vi "LoadData.vi"   [LabVIEW 2019]
uses:
  20200219Virbtion/Typedef/State.ctl
  LLB/Commonly VI/Ctrl/IDLevel.ctl
  Class/Main Process Class/MPC_VirbVision/Panel RefGlb.vi
  LLB/Commonly VI/Load Glb.vi
types:
  T1 = enum16{"initial", "save", "load", "write", "read"}
  T2 = enum16{"Initial", "Load", "Save", "Read", "WriteSpeed", "WritePoint"}
  T3 = enum8{"Enabled", "Disabled", "Disabled and Grayed Out"}
  T4 = typedef "IDLevel.ctl" = enum16{"Administrator", "Engineer", "Operator", "LogIn/Out"}
  T5 = typedef "State.ctl" = enum16{"Initalize", "Idle", "Update", "Channel1", "Channel2", "Channel3", "Channel4", "Channel1 Sample", "Channel2 Sample", "Channel3 Sample", "Channel4 Sample", "Waveform", "DAQ Rate", "ModelList", "Add", "Remove", "Set Time", "Test", "Start Time", "Check Time", "Save", "Frontward", "Leftward", "Backward", "Rightward", "Stop", "Center", "Bump", "Add Project", "Remove Project", "Project List", "Project Name", "Project OK", "Response", "Exit"}
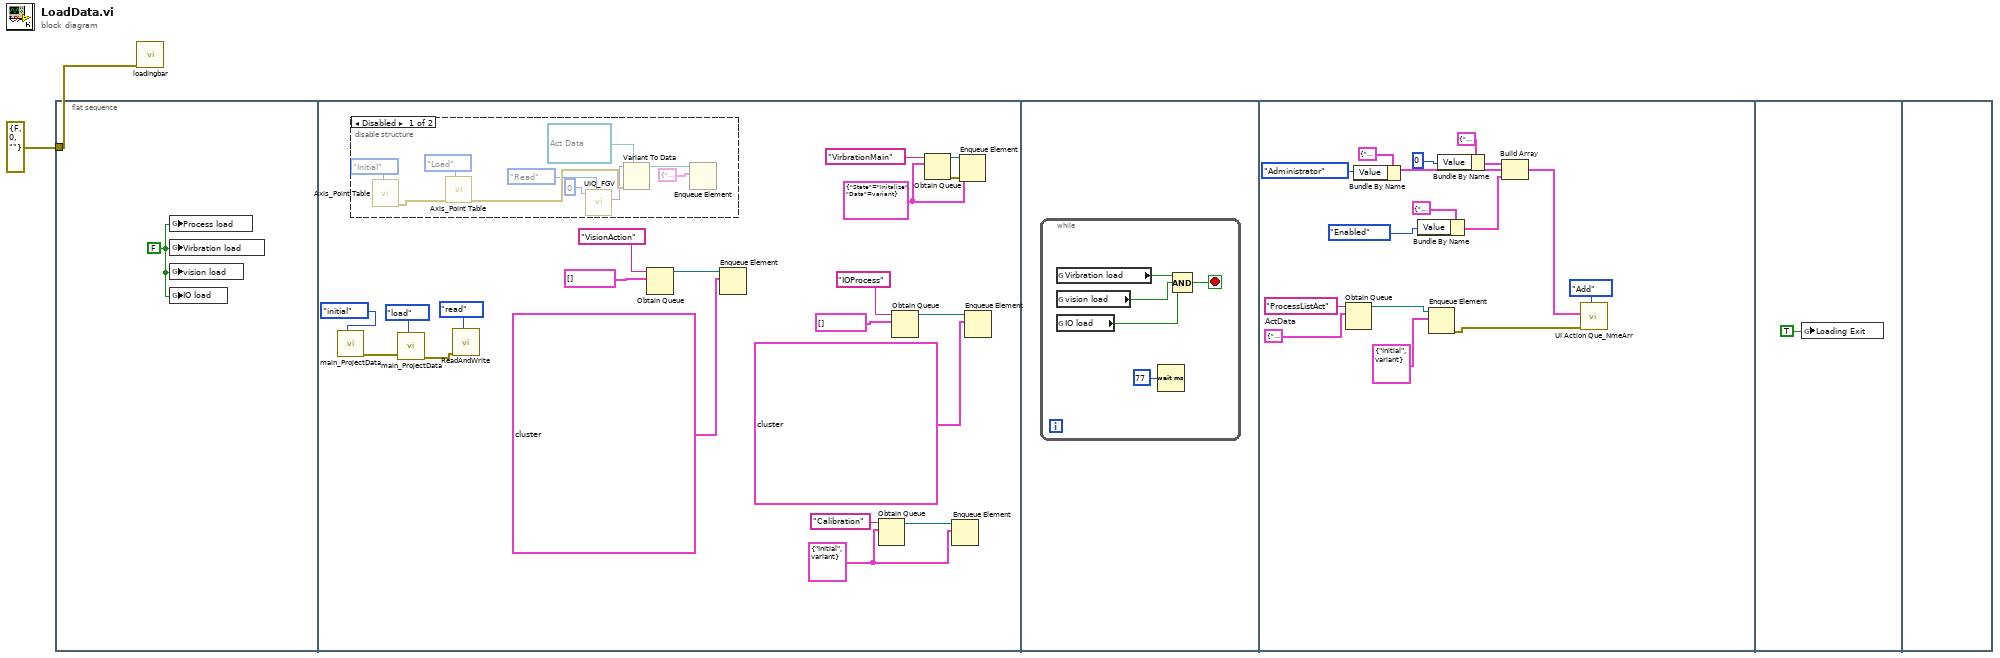
[diagram p0: block diagram]
diagram:
  w1 = errorcluster {"status"=FALSE, "code"=0, "source"=""} ("error constant")
  n1 = flat-sequence {
    tunnel: w1 -> [_]
    frame #0 {
      w2 = FALSE ("IO load")
      n2 = global write "Panel RefGlb.vi" "Process load"(w2) -> ()
      n3 = global write "Panel RefGlb.vi" "Virbration load"(w2) -> ()
      n4 = global write "Panel RefGlb.vi" "vision load"(w2) -> ()
      n5 = global write "Panel RefGlb.vi" "IO load"(w2) -> ()
    }
    frame #1 {
      w19 = cluster{"State":T5, "Data":variant} {"State"=enum."Initalize", "Data"=variant}
      w20 = cluster{"Action":string, "Varient":variant} {"Action"="Initial", "Varient"=variant} ("element")
      n6 = call "main_ProjectData.vi"("Enum"=T1."initial") -> ("error out"=w3:errorcluster)  [unwired: 8 in, 2 out]
      n7 = disable-structure shown="Disabled" {
        frame Disabled {
          n8 = call "Axis_Point Table.vi"("Enum"=T2."Initial") -> ("error Out"=w32:errorcluster)  [unwired: 8 in, 2 out]
          n9 = call "Axis_Point Table.vi"("Enum"=T2."Load", "error In"=w32) -> ("error Out"=w30:errorcluster)  [unwired: 7 in, 2 out]
          n10 = call "UIQ_FGV.vi"("Enum"=enum16{"Initial", "Write", "Read"}."Read", "Index"=0) -> ("DataOut"=w26:variant)  [unwired: 9 in]
          n11 = Variant To Data(error in=w30, type=refnum<queue> refnum ("Axis Q"), Variant=w26) -> (data=w27:refnum<queue>)  [unwired: 1 out]
          n12 = Enqueue Element(queue=w27, element=cluster{"Action":string, "Data":variant} {"Action"="LoadParameter", "Data"=variant}) -> ()  [unwired: 2 in, 3 out]
        }
        frame Enabled {
        }
      }
      n13 = call "main_ProjectData.vi"("Enum"=T1."load", "error in"=w3) -> ("error out"=w7:errorcluster)  [unwired: 7 in, 2 out]
      n14 = call "ReadAndWrite.vi"("Enum"=enum16{"initial", "save", "read"}."read", "error in"=w7) -> ()  [unwired: 9 in, 1 out]
      n15 = Obtain Queue(name (unnamed)="VisionAction", element data type=cluster{"Action":string, "Varient":variant}[] []) -> (queue out=w9:refnum<queue>)  [unwired: 3 in, 2 out]
      n16 = Enqueue Element(queue=w9, element=cluster{"Action":string, "Varient":variant}[] [{"Action"="Get Root Path", "Varient"=variant}, {"Action"="Initial Project", "Varient"=variant}, {"Action"="UpdateProjectSet", "Varient"=variant}, {"Action"="UpDateDataToList ROI", "Varient"=variant}, {"Action"="Initial Camera", "Varient"=variant}, {"Action"="loadfinish", "Varient"=variant}]) -> ()  [unwired: 2 in, 3 out]
      n17 = Obtain Queue(name (unnamed)="Calibration", element data type=w20) -> (queue out=w21:refnum<queue>)  [unwired: 3 in, 2 out]
      n18 = Obtain Queue(name (unnamed)="IOProcess", element data type=cluster{"Action":string, "Varient":variant}[] []) -> (queue out=w13:refnum<queue>)  [unwired: 3 in, 2 out]
      n19 = Obtain Queue(name (unnamed)="VirbrationMain", element data type=w19) -> (queue out=w17:refnum<queue>, error out=w16:errorcluster)  [unwired: 3 in, 1 out]
      n20 = Enqueue Element(queue=w21, element=w20) -> ()  [unwired: 2 in, 3 out]
      n21 = Enqueue Element(queue=w17, element=w19, error in (no error)=w16) -> ()  [unwired: 1 in, 3 out]
      n22 = Enqueue Element(queue=w13, element=cluster{"Action":string, "Varient":variant}[] [{"Action"="Get Root Path", "Varient"=variant}, {"Action"="Initial Project", "Varient"=variant}, {"Action"="UpdateProjectSet", "Varient"=variant}, {"Action"="Initial IOName", "Varient"=variant}, {"Action"="loadfinish", "Varient"=variant}]) -> ()  [unwired: 2 in, 3 out]
    }
    frame #2 {
      n23 = while {
        stop <- w34 stop-if-true
        n24 = global read "Panel RefGlb.vi" "Virbration load"() -> (w37:bool)
        n25 = global read "Panel RefGlb.vi" "vision load"() -> (w36:bool)
        n26 = global read "Panel RefGlb.vi" "IO load"() -> (w35:bool)
        n27 = Wait (ms)(milliseconds to wait=u32 77) -> ()  [unwired: 1 out]
        n28 = Compound Arithmetic op=AND(w37, w36, w35) -> (w34:bool)
      }
    }
    frame #3 {
      w52 = cluster{"Action":string, "Data":variant} {"Action"="", "Data"=variant}  # ActData
      n29 = Obtain Queue(name (unnamed)="ProcessListAct", element data type=w52) -> (queue out=w50:refnum<queue>)  [unwired: 3 in, 2 out]
      n30 = Bundle By Name(cluster=cluster{"Action":string, "Value":variant} {"Action"="ChangeMenuBar", "Value"=variant} ("UI Action"), "Value"=IDLevel."Administrator" ("Entry Level")) -> (w41:cluster{"Action":string, "Value":variant})
      n31 = Bundle By Name(cluster=cluster{"Action":string, "Value":variant} {"Action"="AutorunEnable", "Value"=variant} ("UI Action"), "Value"=T3."Enabled" ("Disabled")) -> (w39:cluster{"Action":string, "Value":variant})
      n32 = Enqueue Element(queue=w50, element=cluster{"Action":string, "Data":variant} {"Action"="Initial", "Data"=variant}) -> (error out=w45:errorcluster)  [unwired: 2 in, 2 out]
      n33 = Bundle By Name(cluster=cluster{"Action":string, "Value":variant} {"Action"="ChangePage", "Value"=variant} ("UI Action"), "Value"=0) -> (w47:cluster{"Action":string, "Value":variant})
      n34 = Build Array(w47, w41, w39) -> (w46:cluster{"Action":string, "Value":variant}[])
      n35 = call "UI Action Que_NmeArr.vi"("Action"=enum16{"Initial", "Add", "Release"}."Add", "error in (no error)"=w45, "UI Process"=w46) -> ()  [unwired: 7 in, 2 out]
    }
    frame #4 {
      n36 = global write "Load Glb.vi" "Loading Exit"(TRUE ("Loading Exit")) -> ()
    }
    frame #5 {
    }
  }
  n37 = call "loadingbar.vi"("error in"=w1) -> ()  [unwired: 10 in, 1 out]
